vi "Process.vi"(8 "error in":errorcluster, 11 "Plugin in":refnum<class "CSV Export.lvclass">) -> (0 "error out":errorcluster, 3 "Plugin out":refnum<class "CSV Export.lvclass">)   [LabVIEW 2022 SP3, in "CSV Export.lvlib" / "CSV Export.lvclass"]
uses:
  CSV Export.lvclass
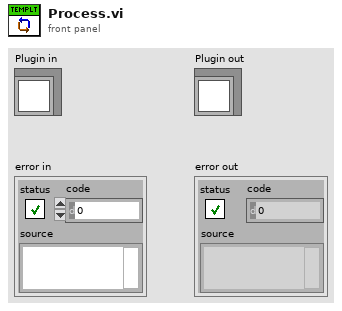
[diagram p1: front panel]
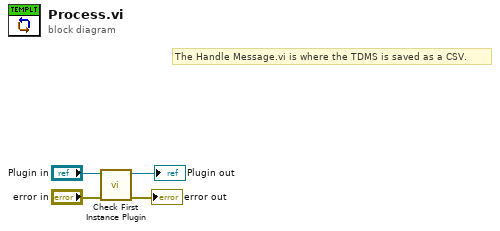
[diagram p0: block diagram]
diagram:
  # "The Handle Message.vi is where the TDMS is saved as a CSV."
  n1 = call "Check First Instance Plugin.vi"("error in (no error)"="error in", "Plugin in"="Plugin in") -> ("error out"=→"error out":errorcluster, "Plugin out"=→"Plugin out":refnum<class "CSV Export.lvclass">)  [unwired: 8 in]
